vi "initialise.vi"(8 "error in (no error)":errorcluster, 10 "folder path":path, 11 "notebook control ref":refnum<vi>) -> (0 "error out":errorcluster, 3 "Notebook out":refnum<class "Notebook.lvclass">)   [LabVIEW 2010, in "Notebook.lvclass"]
uses:
  Notebook.lvclass
  Notebook.lvclass/Notebook.ctl
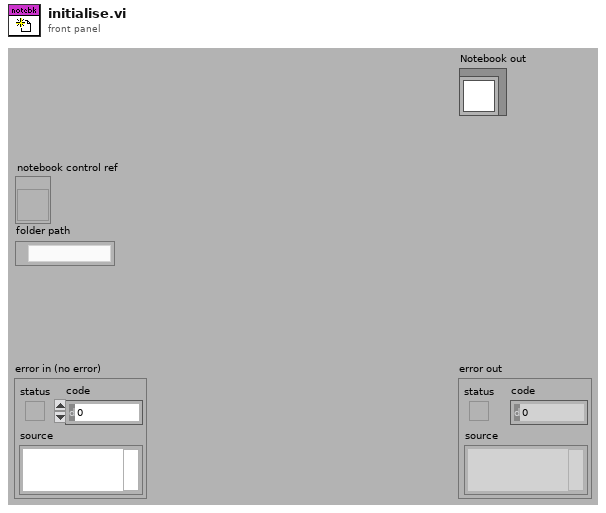
[diagram p1: front panel]
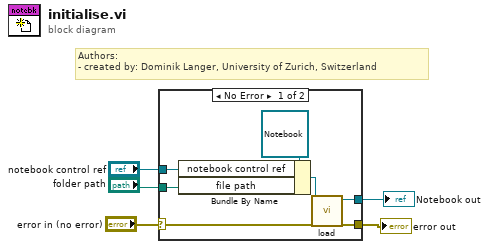
[diagram p0: block diagram]
diagram:
  # "Authors: \n- created by: Dominik Langer, University of Zurich, Switzerland"
  n1 = case shown="No Error" "error in (no error)" {
    selector: "error in (no error)" -> [w11 w13]
    tunnel: [w10 w13] -> w4
    tunnel: [w7 _] -> w3
    tunnel: "notebook control ref" -> [w12 _]
    tunnel: "folder path" -> [w6 _]
    frame No Error {
      n2 = Bundle By Name(cluster=refnum<class "Notebook.lvclass"> refnum ("Notebook.lvclass"), "notebook control ref"=w12, "file path"=w6) -> (w8:refnum<class "Notebook.lvclass">)
      n3 = call "load.vi"("error in (no error)"=w11, "Notebook in"=w8) -> ("error out"=w10:errorcluster, "Notebook out"=w7:refnum<class "Notebook.lvclass">)  [unwired: 8 out]
    }
    frame Error {
    }
  }
  "error out" <- w4
  "Notebook out" <- w3
